vi "ex4-10.vi"   [LabVIEW 2009]
uses:
  <vilib>/NXT/Dual Mode Library/Waits/Wait_Num.vi
  <vilib>/NXT/Dual Mode Library/Motors/MotorOn.vi
  <vilib>/NXT/Dual Mode Library/Motors/MotorReverse.vi
types:
  T1 = typedef "LVHSConnector.ctl" = cluster{"error":errorcluster, "address":string, "NXT #":i32, "Show Error":bool, "Connection":u16}
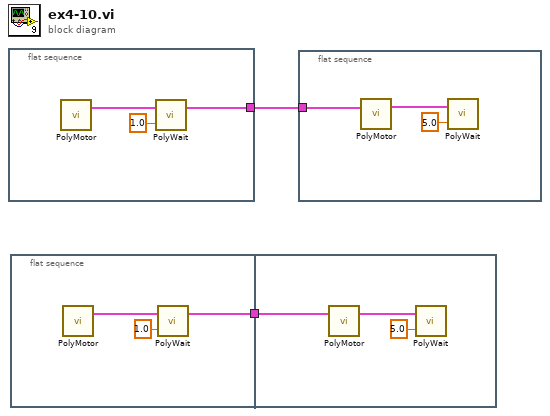
[diagram p0: block diagram]
diagram:
  n1 = flat-sequence {
    tunnel: [w4] -> w2
    frame #0 {
      n2 = call-poly <vilib>:"PolyMotor.vi"() -> ("NXT"=w5:T1)  [unwired: 4 in]
      n3 = call-poly <vilib>:"PolyWait.vi"("Time (1 sec)"=sgl 1.0, "NXT"=w5) -> ("NXT"=w4:T1)  [unwired: 2 in]
    }
  }
  n4 = flat-sequence {
    tunnel: [w7] -> w1
    tunnel: w1 -> [w9]
    frame #0 {
      n5 = call-poly <vilib>:"PolyMotor.vi"() -> ("NXT"=w8:T1)  [unwired: 4 in]
      n6 = call-poly <vilib>:"PolyWait.vi"("Time (1 sec)"=sgl 1.0, "NXT"=w8) -> ("NXT"=w7:T1)  [unwired: 2 in]
    }
    frame #1 {
      n7 = call-poly <vilib>:"PolyMotor.vi"("NXT"=w9) -> ("NXT"=w11:T1)  [unwired: 3 in]
      n8 = call-poly <vilib>:"PolyWait.vi"("Time (1 sec)"=sgl 5.0, "NXT"=w11) -> ()  [unwired: 2 in, 1 out]
    }
  }
  n9 = flat-sequence {
    tunnel: w2 -> [w14]
    frame #0 {
      n10 = call-poly <vilib>:"PolyMotor.vi"("NXT"=w14) -> ("NXT"=w13:T1)  [unwired: 3 in]
      n11 = call-poly <vilib>:"PolyWait.vi"("Time (1 sec)"=sgl 5.0, "NXT"=w13) -> ()  [unwired: 2 in, 1 out]
    }
  }
